vi "Device Clear.vi"(8 "error in (no error)":errorcluster, 11 "VISA Resource Name":refnum<visa-resource-name>) -> (0 "error out":errorcluster, 3 "VISA Resource Out":refnum<visa-resource-name>)   [LabVIEW 2020, in "Agilent 34401.lvlib"]
doc: "Device clear is an IEEE-488 low-level bus message used to halt measurements in progress.\n\nDevice clear performs the following actions:\nAll measurements in progress are aborted.\nThe multimeter returns to the trigger idle state.\nThe multimeter’s input and output buffers are cleared.\nThe multimeter is prepared to accept a new command string.\n\nDevice Clear does <B>not</B>:\nClear the multimeter's error queue\nClear the multimeter's internal memory buffer."
uses:
  <instrlib>/Agilent 34401/Agilent 34401.lvlib
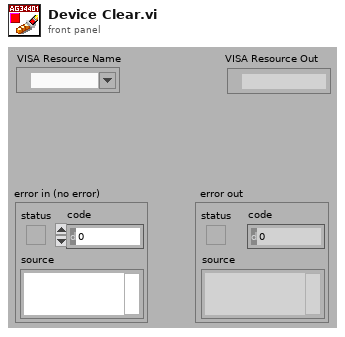
[diagram p1: front panel]
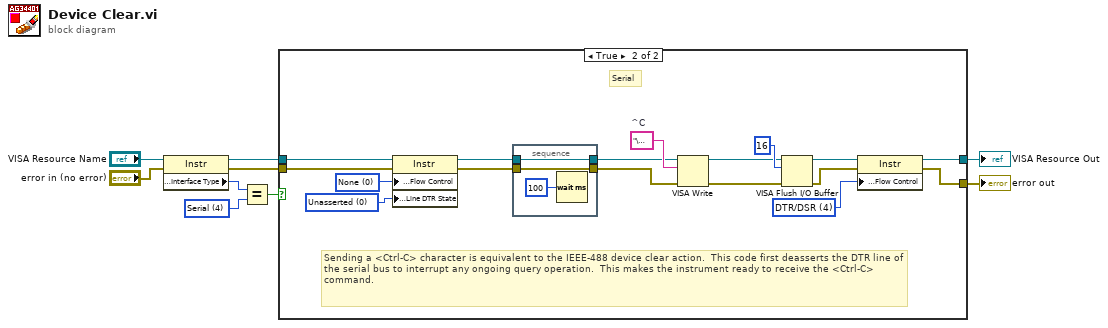
[diagram p0: block diagram]
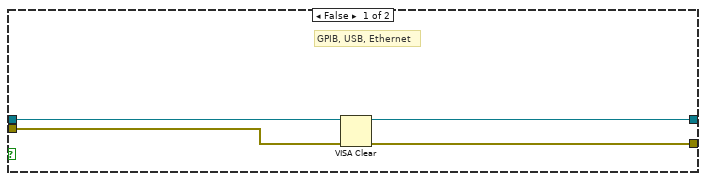
[diagram p2: hidden frame]
diagram:
  w1 = u16 4 items=["GPIB"=1, "VXI"=2, "GPIB-VXI"=3, "Serial"=4, "PXI"=5, "TCPIP"=6, "USB"=7] ("Interface Information:Interface Type")
  n1 = property on="Property Node" class="Instr"(reference="VISA Resource Name", error in="error in (no error)") -> (reference out=w9:refnum<visa-resource-name>, error out=w5:errorcluster, "Interface Information:Interface Type"=w4:u16)
  n2 = Equal?(x=w4, y=w1) -> (x = y?=w8:bool)
  n3 = case shown="True" w8 {
    tunnel: w5 -> [w10 w29]
    tunnel: [w12 w26] -> w3
    tunnel: [w11 w25] -> w2
    tunnel: w9 -> [w13 w30]
    frame False {
      # "GPIB, USB, Ethernet"
      n4 = VISA Clear(VISA resource name=w13, error in (no error)=w10) -> (VISA resource name out=w12:refnum<visa-resource-name>, error out=w11:errorcluster)
    }
    frame True {
      w27 = u16 4 items=["None"=0, "XON/XOFF"=1, "RTS/CTS"=2, "DTR/DSR"=4] ("Serial Settings:Serial Flow Control")
      w20 = u16 0 items=["None"=0, "XON/XOFF"=1, "RTS/CTS"=2, "DTR/DSR"=4] ("Serial Settings:Serial Flow Control")
      w28 = "\u0003"  # ^C
      w21 = i16 0 items=["Unknown"=-1, "Unasserted"=0, "Asserted"=1] ("Modem Line Settings:Line DTR State")
      # "Sending a <Ctrl-C> character is equivalent to the IEEE-488 device clear action.  This code first deasserts the DTR line of the serial bus to interrupt any ongoing query operation.  This makes the instrument ready to receive the <Ctrl-C> command."
      # "Serial"
      n5 = property on="Property Node" class="Instr"(reference=w30, error in=w29, "Serial Settings:Flow Control"=w20, "Serial Settings:Modem Line Settings:Line DTR State"=w21) -> (reference out=w24:refnum<visa-resource-name>, error out=w23:errorcluster)
      n6 = stacked-sequence {
        tunnel: [w32] -> w19
        tunnel: w24 -> [w32]
        tunnel: [w31] -> w18
        tunnel: w23 -> [w31]
        frame #0 {
          n7 = Wait (ms)(milliseconds to wait=u32 100) -> ()  [unwired: 1 out]
        }
      }
      n8 = VISA Write(VISA resource name=w19, write buffer=w28, error in (no error)=w18) -> (VISA resource name out=w15:refnum<visa-resource-name>, error out=w14:errorcluster)  [unwired: 1 out]
      n9 = VISA Flush I/O Buffer(VISA resource name=w15, mask (16)=u16 16, error in (no error)=w14) -> (VISA resource name out=w17:refnum<visa-resource-name>, error out=w16:errorcluster)
      n10 = property on="Property Node" class="Instr"(reference=w17, error in=w16, "Serial Settings:Flow Control"=w27) -> (reference out=w26:refnum<visa-resource-name>, error out=w25:errorcluster)
    }
  }
  "VISA Resource Out" <- w3
  "error out" <- w2
